vi "CH0_write_byte_data_and_sign_into_mem_no_g_Rev02.vi"(0 "MB data":u8, 1 "UB data":u8, 3 "Sign addrss 8 byte":string, 4 "USB Interface Name":refnum<visa-resource-name>="COM3", 5 "HB data":u8, 7 "LB data":u8, 8 "MB addrss 8 byte":string, 9 "HB addrss 8 byte":string, 11 "LB addrss 8 byte":string, 12 "Sign data 3 byte":dbl, 13 "WRITE DATA":bool, 14 "Input buffer size":u32=16384, 16 "UB addrss 8 byte":string, 17 "error in (no error)":errorcluster, 23 "Enable memory wright":bool) -> (10 "Reply 1":string, 18 "Reply 2":string, 20 "MB data 3 byte":string, 21 "UB data 3 byte":string, 22 "Reply 3":string, 24 "error out":errorcluster, 25 "HB data 3 byte":string, 26 "Reply 4":string, 27 "LB data 3 byte":string)   [LabVIEW 2012]
panel:
  out "Sent command":string
  out "T command Bytes sent 5":dbl
  out "T command Bytes sent 4":dbl
  out "T command Bytes sent 3":dbl
  out "T command Bytes sent 2":dbl
  out "T command Bytes sent":dbl
  out "First 'T' Number of bytes written":dbl
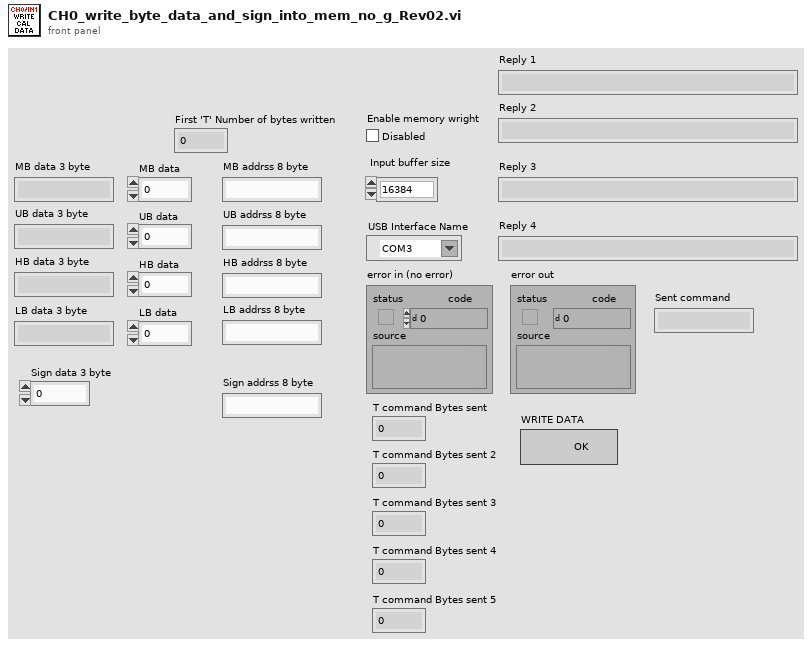
[diagram p1: front panel]
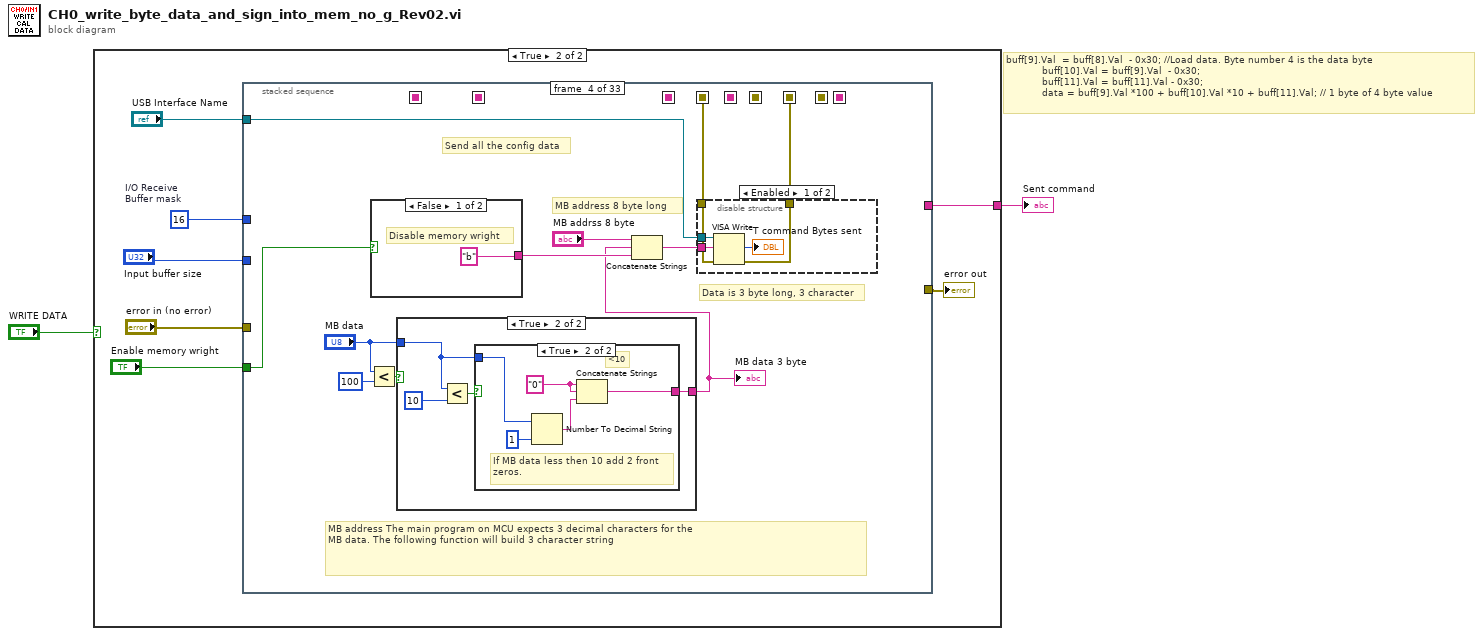
[diagram p0: block diagram]
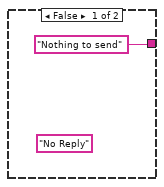
[diagram p2: hidden frame]
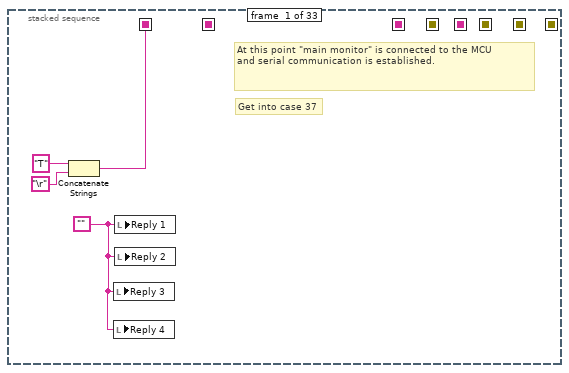
[diagram p3: hidden frame]
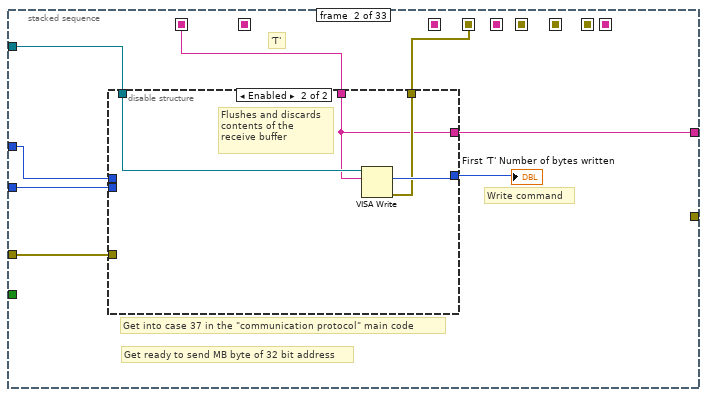
[diagram p4: hidden frame]
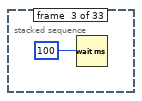
[diagram p6: hidden frame]
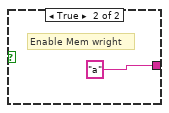
[diagram p7: hidden frame]
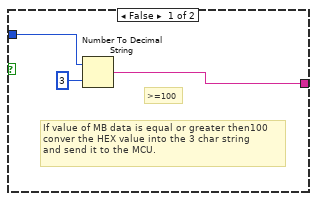
[diagram p8: hidden frame]
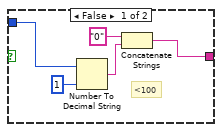
[diagram p9: hidden frame]
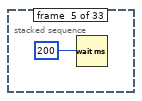
[diagram p11: hidden frame]
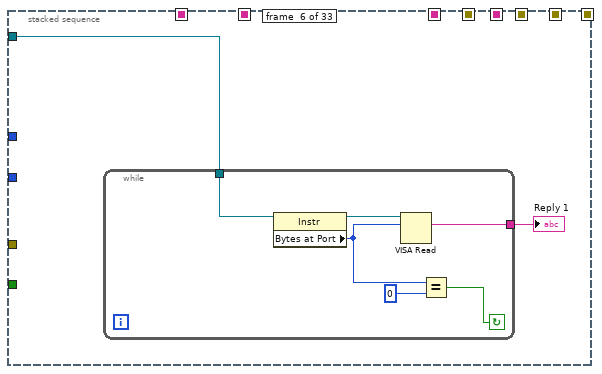
[diagram p12: hidden frame]
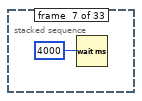
[diagram p13: hidden frame]
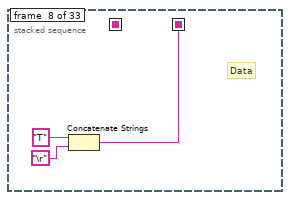
[diagram p14: hidden frame]
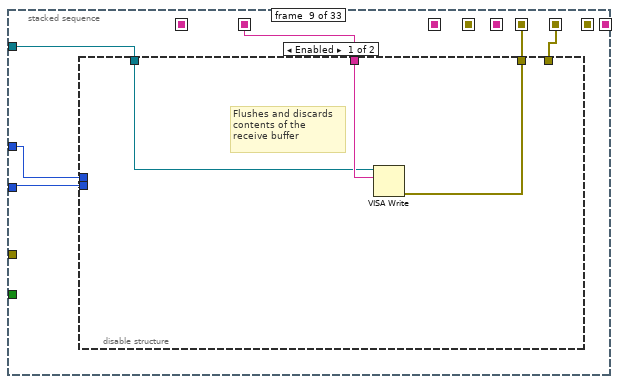
[diagram p15: hidden frame]
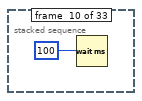
[diagram p17: hidden frame]
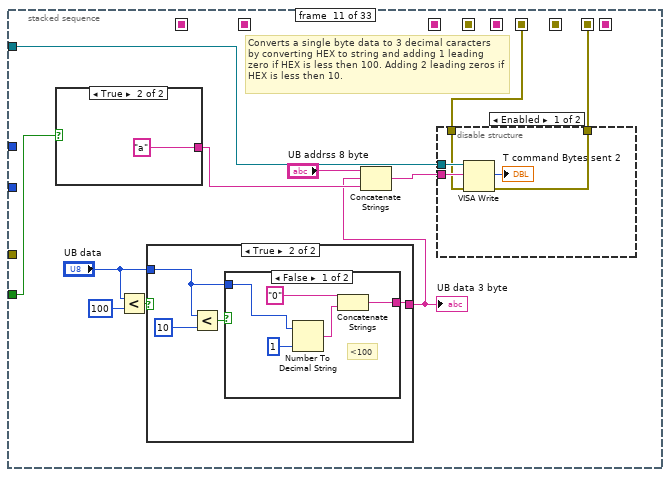
[diagram p18: hidden frame]
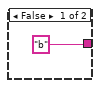
[diagram p19: hidden frame]
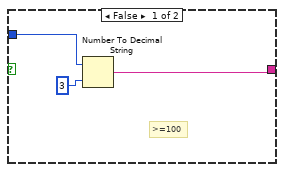
[diagram p20: hidden frame]
diagram:
  # "buff[9].Val  = buff[8].Val  - 0x30; //Load data. Byte number 4 is the data byte           \n            buff[10].Val = buff[9].Val  - 0x30;           \n            buff[11].Val = buff[11].Val - 0x30;               \n            data = buff[9].Val *100 + buff[10].Val *10 + buff[11].Val; // 1 byte of 4 byte value"
  n1 = case shown="True" "WRITE DATA" {
    tunnel: ["Nothing to send" w4] -> w1
    frame False {
      (unwired) "No Reply"
    }
    frame True {
      w8 = u16 16  # I/O Receive Buffer mask
      n2 = stacked-sequence {
        seq-local: [w12 _ _ _ _ _ _ _ _ _ _ _ _ _ _ _ _ _ _ _ _ _ _ _ _ _ _ _ _ _ _ _ _] -> [_ w19 _ _ _ _ _ _ _ _ _ _ _ _ _ _ _ _ _ _ _ _ _ _ _ _ _ _ _ _ _ _ _]
        seq-local: [_ _ _ _ _ _ _ w73 _ _ _ _ _ _ _ _ _ _ _ _ _ _ _ _ _ _ _ _ _ _ _ _ _] -> [_ _ _ _ _ _ _ _ w78 _ _ _ _ _ _ _ _ _ _ _ _ _ _ _ _ _ _ _ _ _ _ _ _]
        seq-local: [_ _ _ _ _ _ _ _ _ _ _ _ _ _ w131 _ _ _ _ _ _ _ _ _ _ _ _ _ _ _ _ _ _] -> [_ _ _ _ _ _ _ _ _ _ _ _ _ _ _ w135 _ _ _ _ _ _ _ _ _ _ _ _ _ _ _ _ _]
        seq-local: [_ _ _ _ _ _ _ _ _ _ _ _ _ _ _ _ _ _ _ _ _ w184 _ _ _ _ _ _ _ _ _ _ _] -> [_ _ _ _ _ _ _ _ _ _ _ _ _ _ _ _ _ _ _ _ _ _ w187 _ _ _ _ _ _ _ _ _ _]
        seq-local: [_ w18 _ _ _ _ _ _ _ _ _ _ _ _ _ _ _ _ _ _ _ _ _ _ _ _ _ _ _ _ _ _ _] -> [_ _ _ w34 _ _ _ _ _ _ _ _ _ _ _ _ _ _ _ _ _ _ _ _ _ _ _ _ _ _ _ _ _]
        seq-local: [_ _ _ w33 _ _ _ _ _ _ _ _ _ _ _ _ _ _ _ _ _ _ _ _ _ _ _ _ _ _ _ _ _] -> [_ _ _ _ _ _ _ _ w77 _ _ _ _ _ _ _ _ _ _ _ _ _ _ _ _ _ _ _ _ _ _ _ _]
        seq-local: [_ _ _ _ _ _ _ _ w76 _ _ _ _ _ _ _ _ _ _ _ _ _ _ _ _ _ _ _ _ _ _ _ _] -> [_ _ _ _ _ _ _ _ _ _ w92 _ _ _ _ _ _ _ _ _ _ _ _ _ _ _ _ _ _ _ _ _ _]
        seq-local: [_ _ _ _ _ _ _ _ _ _ w91 _ _ _ _ _ _ _ _ _ _ _ _ _ _ _ _ _ _ _ _ _ _] -> [_ _ _ _ _ _ _ _ _ _ _ _ _ _ _ w134 _ _ _ _ _ _ _ _ _ _ _ _ _ _ _ _ _]
        seq-local: [_ _ _ _ _ _ _ _ _ _ _ _ _ _ _ _ _ _ _ _ _ _ _ _ _ _ _ _ w239 _ _ _ _] -> [_ _ _ _ _ _ _ _ _ _ _ _ _ _ _ _ _ _ _ _ _ _ _ _ _ _ _ _ _ w242 _ _ _]
        tunnel: "USB Interface Name" -> [_ w22 _ w37 _ w65 _ _ w81 _ w93 _ w123 _ _ w138 _ w148 _ w176 _ _ w191 _ w202 _ w231 _ _ w246 _ w259 _]
        tunnel: "error in (no error)" -> [_ w21 _ _ _ _ _ _ _ _ _ _ _ _ _ _ _ _ _ _ _ _ w189 _ _ _ _ _ _ w243 _ _ _]
        tunnel: "Input buffer size" -> [_ w20 _ _ _ _ _ _ w80 _ _ _ _ _ _ w136 _ _ _ _ _ _ w190 _ _ _ _ _ _ w244 _ _ _]
        tunnel: w8 -> [_ w16 _ _ _ _ _ _ w79 _ _ _ _ _ _ w137 _ _ _ _ _ _ w188 _ _ _ _ _ _ w245 _ _ _]
        tunnel: [_ _ _ _ _ _ _ _ _ _ _ _ _ _ _ _ _ _ _ _ _ _ _ _ w201 _ _ _ _ _ _ _ _] -> w7
        tunnel: "Enable memory wright" -> [_ _ _ w31 _ _ _ _ _ _ w88 _ _ _ _ _ _ w146 _ _ _ _ _ _ w199 _ _ _ _ _ _ w251 _]
        tunnel: [_ w15 _ _ _ _ _ _ _ _ _ _ _ _ _ _ _ _ _ _ _ _ _ _ _ _ _ _ _ _ _ _ _] -> w4
        frame #0 {
          w11 = ""
          # "At this point \"main monitor\" is connected to the MCU\nand serial communication is established."
          # "Get into case 37"
          n3 = Concatenate Strings("T", "\r") -> (w12:string)
          n4 = local write "Reply 3"(w11) -> ()
          n5 = local write "Reply 4"(w11) -> ()
          n6 = local write "Reply 1"(w11) -> ()
          n7 = local write "Reply 2"(w11) -> ()
        }
        frame #1 {
          # "Get ready to send MB byte of 32 bit address"
          # "'T'"
          # "Get into case 37 in the \"communication protocol\" main code"
          # "Write command"
          n8 = disable-structure shown="Enabled" {
            disable-tunnel: w20 -> [_ _]
            disable-tunnel: w19 -> [_ w23]
            disable-tunnel: w22 -> [_ w24]
            disable-tunnel: w21 -> [_ _]
            disable-tunnel: [_ w26] -> w17
            disable-tunnel: [_ w25] -> w18
            disable-tunnel: w16 -> [_ _]
            disable-tunnel: [_ w23] -> w15
            frame Disabled {
            }
            frame Enabled {
              # "Flushes and discards \ncontents of the \nreceive buffer"
              n9 = VISA Write(VISA resource name=w24, write buffer=w23) -> (return count=w26:u32, error out=w25:errorcluster)  [unwired: 1 in, 1 out]
            }
          }
          "First 'T' Number of bytes written" <- w17
        }
        frame #2 {
          n10 = Wait (ms)(milliseconds to wait=100) -> ()  [unwired: 1 out]
        }
        frame #3 {
          # "Send all the config data"
          # "MB address 8 byte long"
          # "Data is 3 byte long, 3 character"
          # "MB address The main program on MCU expects 3 decimal characters for the \nMB data. The following function will build 3 character string"
          n11 = Less?(x="MB data", y=100) -> (x < y?=w36:bool)
          n12 = case shown="False" w31 {
            tunnel: ["b" "a"] -> w30
            frame False {
              # "Disable memory wright"
            }
            frame True {
              # "Enable Mem wright"
            }
          }
          n13 = case shown="True" w36 {
            tunnel: [w43 w44] -> w28
            tunnel: "MB data" -> [w41 w45]
            frame False {
              # "If value of MB data is equal or greater then100\nconver the HEX value into the 3 char string \nand send it to the MCU."
              # ">=100"
              n14 = Number To Decimal String(number=w41, width (-)=3) -> (decimal integer string=w43:string)
            }
            frame True {
              n15 = Less?(x=w45, y=10) -> (x < y?=w47:bool)
              n16 = case shown="True" w47 {
                tunnel: w45 -> [w50 w53]
                tunnel: [w49 w54] -> w44
                frame False {
                  # "<100"
                  n17 = Number To Decimal String(number=w50, width (-)=1) -> (decimal integer string=w51:string)
                  n18 = Concatenate Strings("0", w51) -> (w49:string)
                }
                frame True {
                  w55 = "0"
                  # "If MB data less then 10 add 2 front\nzeros."
                  # "<10"
                  n19 = Number To Decimal String(number=w53, width (-)=1) -> (decimal integer string=w56:string)
                  n20 = Concatenate Strings(w55, w55, w56) -> (w54:string)
                }
              }
            }
          }
          "MB data 3 byte" <- w28
          n21 = Concatenate Strings("MB addrss 8 byte", w28, w30) -> (w38:string)
          n22 = disable-structure shown="Enabled" {
            disable-tunnel: w38 -> [w61 _]
            disable-tunnel: w37 -> [w60 _]
            disable-tunnel: w34 -> [w59 _]
            disable-tunnel: [w58 _] -> w33
            frame Enabled {
              n23 = VISA Write(VISA resource name=w60, write buffer=w61, error in (no error)=w59) -> (return count=→"T command Bytes sent":u32, error out=w58:errorcluster)  [unwired: 1 out]
            }
            frame Disabled {
            }
          }
        }
        frame #4 {
          n24 = Wait (ms)(milliseconds to wait=200) -> ()  [unwired: 1 out]
        }
        frame #5 {
          n25 = while {
            tunnel: w65 -> [w67]
            tunnel: [w66] -> w64
            stop <- w68 continue-if-true
            n26 = property class="Instr"(reference=w67) -> (reference out=w71:refnum<visa-resource-name>, "Bytes at Port"=w70:u32)  [unwired: 1 in, 1 out]
            n27 = VISA Read(VISA resource name=w71, byte count=w70) -> (read buffer=w66:string)  [unwired: 1 in, 3 out]
            n28 = Equal?(x=w70, y=0) -> (x = y?=w68:bool)
          }
          "Reply 1" <- w64
        }
        frame #6 {
          n29 = Wait (ms)(milliseconds to wait=4000) -> ()  [unwired: 1 out]
        }
        frame #7 {
          # "Data"
          n30 = Concatenate Strings("T", "\r") -> (w73:string)
        }
        frame #8 {
          n31 = disable-structure shown="Enabled" {
            disable-tunnel: w81 -> [w82 _]
            disable-tunnel: w80 -> [_ _]
            disable-tunnel: w79 -> [_ _]
            disable-tunnel: w78 -> [w84 _]
            disable-tunnel: w77 -> [_ _]
            disable-tunnel: [w83 _] -> w76
            frame Enabled {
              # "Flushes and discards \ncontents of the \nreceive buffer"
              n32 = VISA Write(VISA resource name=w82, write buffer=w84) -> (error out=w83:errorcluster)  [unwired: 1 in, 2 out]
            }
            frame Disabled {
            }
          }
        }
        frame #9 {
          n33 = Wait (ms)(milliseconds to wait=100) -> ()  [unwired: 1 out]
        }
        frame #10 {
          # "Converts a single byte data to 3 decimal caracters\nby converting HEX to string and adding 1 leading zero if HEX is less then 100. Adding 2 leading zeros if HEX is less then 10."
          n34 = case shown="True" w88 {
            tunnel: ["b" "a"] -> w89
            frame False {
            }
            frame True {
            }
          }
          n35 = Less?(x="UB data", y=100) -> (x < y?=w95:bool)
          n36 = case shown="True" w95 {
            tunnel: [w101 w102] -> w86
            tunnel: "UB data" -> [w99 w103]
            frame False {
              # ">=100"
              n37 = Number To Decimal String(number=w99, width (-)=3) -> (decimal integer string=w101:string)
            }
            frame True {
              n38 = Less?(x=w103, y=10) -> (x < y?=w105:bool)
              n39 = case shown="False" w105 {
                tunnel: w103 -> [w107 w111]
                tunnel: [w106 w112] -> w102
                frame False {
                  # "<100"
                  n40 = Number To Decimal String(number=w107, width (-)=1) -> (decimal integer string=w108:string)
                  n41 = Concatenate Strings("0", w108) -> (w106:string)
                }
                frame True {
                  w113 = "0"
                  # "<10"
                  n42 = Number To Decimal String(number=w111, width (-)=1) -> (decimal integer string=w114:string)
                  n43 = Concatenate Strings(w113, w113, w114) -> (w112:string)
                }
              }
            }
          }
          "UB data 3 byte" <- w86
          n44 = Concatenate Strings("UB addrss 8 byte", w86, w89) -> (w96:string)
          n45 = disable-structure shown="Enabled" {
            disable-tunnel: w96 -> [w119 _]
            disable-tunnel: w93 -> [w118 _]
            disable-tunnel: w92 -> [w117 _]
            disable-tunnel: [w116 _] -> w91
            frame Enabled {
              n46 = VISA Write(VISA resource name=w118, write buffer=w119, error in (no error)=w117) -> (return count=→"T command Bytes sent 2":u32, error out=w116:errorcluster)  [unwired: 1 out]
            }
            frame Disabled {
            }
          }
        }
        frame #11 {
          n47 = Wait (ms)(milliseconds to wait=200) -> ()  [unwired: 1 out]
        }
        frame #12 {
          n48 = while {
            tunnel: w123 -> [w125]
            tunnel: [w124] -> w122
            stop <- w126 continue-if-true
            n49 = property class="Instr"(reference=w125) -> (reference out=w129:refnum<visa-resource-name>, "Bytes at Port"=w128:u32)  [unwired: 1 in, 1 out]
            n50 = VISA Read(VISA resource name=w129, byte count=w128) -> (read buffer=w124:string)  [unwired: 1 in, 3 out]
            n51 = Equal?(x=w128, y=0) -> (x = y?=w126:bool)
          }
          "Reply 2" <- w122
        }
        frame #13 {
          n52 = Wait (ms)(milliseconds to wait=4000) -> ()  [unwired: 1 out]
        }
        frame #14 {
          n53 = Concatenate Strings("T", "\r") -> (w131:string)
        }
        frame #15 {
          n54 = disable-structure shown="Enabled" {
            disable-tunnel: w138 -> [w139 _]
            disable-tunnel: w137 -> [_ _]
            disable-tunnel: w136 -> [_ _]
            disable-tunnel: w135 -> [w140 _]
            disable-tunnel: w134 -> [_ _]
            frame Enabled {
              # "Flushes and discards \ncontents of the \nreceive buffer"
              n55 = VISA Write(VISA resource name=w139, write buffer=w140) -> ()  [unwired: 1 in, 3 out]
            }
            frame Disabled {
            }
          }
        }
        frame #16 {
          n56 = Wait (ms)(milliseconds to wait=100) -> ()  [unwired: 1 out]
        }
        frame #17 {
          # "Converts a single byte data to 3 decimal caracters\nby converting HEX to string and adding 1 leading zero if HEX is less then 100. Adding 2 leading zeros if HEX is less then 10."
          n57 = case shown="True" w146 {
            tunnel: ["b" "a"] -> w145
            frame False {
            }
            frame True {
            }
          }
          n58 = Less?(x="HB data", y=100) -> (x < y?=w150:bool)
          n59 = case shown="True" w150 {
            tunnel: [w156 w157] -> w142
            tunnel: "HB data" -> [w154 w158]
            frame False {
              # ">=100"
              n60 = Number To Decimal String(number=w154, width (-)=3) -> (decimal integer string=w156:string)
            }
            frame True {
              n61 = Less?(x=w158, y=10) -> (x < y?=w160:bool)
              n62 = case shown="False" w160 {
                tunnel: w158 -> [w162 w166]
                tunnel: [w161 w167] -> w157
                frame False {
                  # "<100"
                  n63 = Number To Decimal String(number=w162, width (-)=1) -> (decimal integer string=w163:string)
                  n64 = Concatenate Strings("0", w163) -> (w161:string)
                }
                frame True {
                  w168 = "0"
                  # "<10"
                  n65 = Number To Decimal String(number=w166, width (-)=1) -> (decimal integer string=w169:string)
                  n66 = Concatenate Strings(w168, w168, w169) -> (w167:string)
                }
              }
            }
          }
          "HB data 3 byte" <- w142
          n67 = Number To Decimal String(number="HB data", width (-)=3) -> ()  [unwired: 1 out]
          n68 = Concatenate Strings("HB addrss 8 byte", w142, w145) -> (w151:string)
          n69 = disable-structure shown="Enabled" {
            disable-tunnel: w151 -> [w172 _]
            disable-tunnel: w148 -> [w171 _]
            frame Enabled {
              n70 = VISA Write(VISA resource name=w171, write buffer=w172) -> (return count=→"T command Bytes sent 3":u32)  [unwired: 1 in, 2 out]
            }
            frame Disabled {
            }
          }
        }
        frame #18 {
          n71 = Wait (ms)(milliseconds to wait=200) -> ()  [unwired: 1 out]
        }
        frame #19 {
          n72 = while {
            tunnel: w176 -> [w178]
            tunnel: [w177] -> w175
            stop <- w179 continue-if-true
            n73 = property class="Instr"(reference=w178) -> (reference out=w182:refnum<visa-resource-name>, "Bytes at Port"=w181:u32)  [unwired: 1 in, 1 out]
            n74 = VISA Read(VISA resource name=w182, byte count=w181) -> (read buffer=w177:string)  [unwired: 1 in, 3 out]
            n75 = Equal?(x=w181, y=0) -> (x = y?=w179:bool)
          }
          "Reply 3" <- w175
        }
        frame #20 {
          n76 = Wait (ms)(milliseconds to wait=4000) -> ()  [unwired: 1 out]
        }
        frame #21 {
          # "Get into case 37"
          n77 = Concatenate Strings("T", "\r") -> (w184:string)
        }
        frame #22 {
          # "Get into case 37 in the communication protocol"
          # "Write command"
          n78 = disable-structure shown="Enabled" {
            disable-tunnel: w190 -> [_ _]
            disable-tunnel: w187 -> [w194 _]
            disable-tunnel: w191 -> [w192 _]
            disable-tunnel: w189 -> [_ _]
            disable-tunnel: [w193 _] -> _
            disable-tunnel: w188 -> [_ _]
            frame Enabled {
              # "Flushes and discards \ncontents of the \nreceive buffer"
              n79 = VISA Write(VISA resource name=w192, write buffer=w194) -> (return count=w193:u32)  [unwired: 1 in, 2 out]
            }
            frame Disabled {
            }
          }
        }
        frame #23 {
          n80 = Wait (ms)(milliseconds to wait=100) -> ()  [unwired: 1 out]
        }
        frame #24 {
          # "The main program on MCU expects 3 decimal characters for the \nMB data. The following function will build 3 character string"
          n81 = case shown="True" w199 {
            tunnel: ["b" "a"] -> w198
            frame False {
            }
            frame True {
              # "Enable memory wright"
            }
          }
          n82 = Number To Decimal String(number="LB data") -> ()  [unwired: 1 in, 1 out]
          n83 = Less?(x="LB data", y=100) -> (x < y?=w204:bool)
          n84 = case shown="True" w204 {
            tunnel: [w210 w211] -> w197
            tunnel: "LB data" -> [w208 w212]
            frame False {
              # ">=100"
              n85 = Number To Decimal String(number=w208, width (-)=3) -> (decimal integer string=w210:string)
            }
            frame True {
              n86 = Less?(x=w212, y=10) -> (x < y?=w214:bool)
              n87 = case shown="True" w214 {
                tunnel: w212 -> [w216 w220]
                tunnel: [w215 w221] -> w211
                frame False {
                  # "<100"
                  n88 = Number To Decimal String(number=w216, width (-)=1) -> (decimal integer string=w217:string)
                  n89 = Concatenate Strings("0", w217) -> (w215:string)
                }
                frame True {
                  w222 = "0"
                  # "<10"
                  n90 = Number To Decimal String(number=w220, width (-)=1) -> (decimal integer string=w223:string)
                  n91 = Concatenate Strings(w222, w222, w223) -> (w221:string)
                }
              }
            }
          }
          "LB data 3 byte" <- w197
          n92 = Concatenate Strings("LB addrss 8 byte", w197, w198) -> (w205:string)
          n93 = disable-structure shown="Enabled" {
            disable-tunnel: w205 -> [w227 _]
            disable-tunnel: w202 -> [w226 _]
            disable-tunnel: [w225 _] -> w201
            frame Enabled {
              n94 = VISA Write(VISA resource name=w226, write buffer=w227) -> (return count=→"T command Bytes sent 4":u32, error out=w225:errorcluster)  [unwired: 1 in, 1 out]
            }
            frame Disabled {
            }
          }
        }
        frame #25 {
          n95 = Wait (ms)(milliseconds to wait=200) -> ()  [unwired: 1 out]
        }
        frame #26 {
          n96 = while {
            tunnel: w231 -> [w233]
            tunnel: [w232] -> w230
            stop <- w234 continue-if-true
            n97 = property class="Instr"(reference=w233) -> (reference out=w237:refnum<visa-resource-name>, "Bytes at Port"=w236:u32)  [unwired: 1 in, 1 out]
            n98 = VISA Read(VISA resource name=w237, byte count=w236) -> (read buffer=w232:string)  [unwired: 1 in, 3 out]
            n99 = Equal?(x=w236, y=0) -> (x = y?=w234:bool)
          }
          "Reply 4" <- w230
        }
        frame #27 {
          n100 = Wait (ms)(milliseconds to wait=4000) -> ()  [unwired: 1 out]
        }
        frame #28 {
          # "Send sign"
          n101 = Concatenate Strings("T", "\r") -> (w239:string)
        }
        frame #29 {
          # "Get into case 37 in the communication protocol"
          # "Write command"
          n102 = disable-structure shown="Enabled" {
            disable-tunnel: w244 -> [_ _]
            disable-tunnel: w242 -> [w249 _]
            disable-tunnel: w246 -> [w247 _]
            disable-tunnel: w243 -> [_ _]
            disable-tunnel: [w248 _] -> _
            disable-tunnel: w245 -> [_ _]
            frame Enabled {
              # "Flushes and discards \ncontents of the \nreceive buffer"
              n103 = VISA Write(VISA resource name=w247, write buffer=w249) -> (return count=w248:u32)  [unwired: 1 in, 2 out]
            }
            frame Disabled {
            }
          }
        }
        frame #30 {
          n104 = Wait (ms)(milliseconds to wait=1000) -> ()  [unwired: 1 out]
        }
        frame #31 {
          w256 = "0"
          # "001 or 000"
          # "<10"
          n105 = case shown="True" w251 {
            tunnel: ["b" "a"] -> w252
            frame False {
            }
            frame True {
            }
          }
          n106 = Number To Decimal String(number="Sign data 3 byte", width (-)=1) -> (decimal integer string=w257:string)
          n107 = Concatenate Strings(w256, w256, w257) -> (w254:string)
          n108 = Concatenate Strings("Sign addrss 8 byte", w254, w252) -> (w260:string)
          n109 = disable-structure shown="Enabled" {
            disable-tunnel: w260 -> [w265 _]
            disable-tunnel: w259 -> [w264 _]
            disable-tunnel: [w263 _] -> _
            frame Enabled {
              n110 = VISA Write(VISA resource name=w264, write buffer=w265) -> (return count=→"T command Bytes sent 5":u32, error out=w263:errorcluster)  [unwired: 1 in, 1 out]
            }
            frame Disabled {
            }
          }
        }
        frame #32 {
          n111 = Wait (ms)(milliseconds to wait=3000) -> ()  [unwired: 1 out]
        }
      }
      "error out" <- w7
    }
  }
  "Sent command" <- w1
